vi "Read Speed Setting.vi"(8 "error in (no error)":errorcluster, 11 "Scientifica XYZ Gen1 in":refnum<class "Scientifica XYZ Gen1.lvclass">) -> (0 "error out":errorcluster, 1 "bytes read":u32, 2 "Speed Setting":string, 3 "Scientifica XYZ Gen1 out":refnum<class "Scientifica XYZ Gen1.lvclass">)   [LabVIEW 2020, in "TranslationStageClassStructure.lvlib" / "Scientifica XYZ Gen1.lvclass"]
uses:
  Scientifica XYZ Gen1.lvclass
  Scientifica XYZ Gen1.lvclass/Scientifica XYZ Gen1.ctl
  Serial Comms/Serial Comms/Serial Comms.lvclass
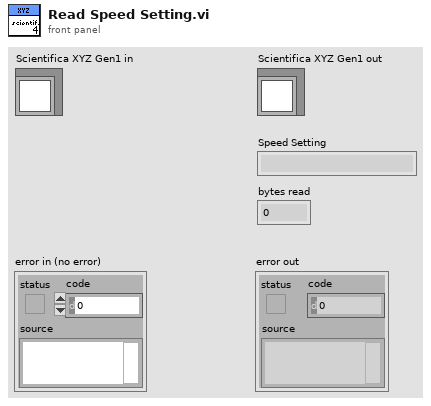
[diagram p1: front panel]
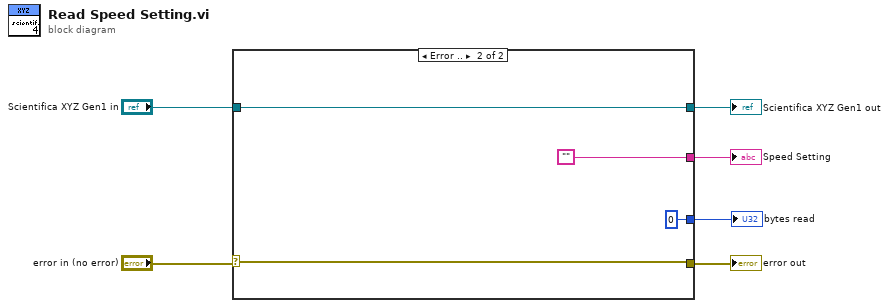
[diagram p0: block diagram]
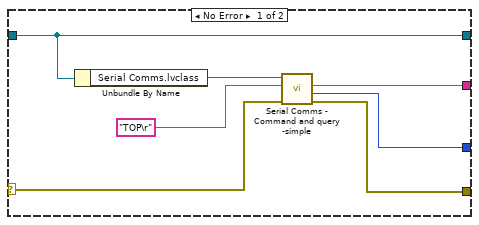
[diagram p2: hidden frame]
diagram:
  n1 = case shown="Error .." "error in (no error)" {
    selector: "error in (no error)" -> [w11 w16]
    tunnel: "Scientifica XYZ Gen1 in" -> [w13 w17]
    tunnel: [w13 w17] -> w4
    tunnel: [w10 w16] -> w3
    tunnel: [w8 ""] -> w2
    tunnel: [w7 u32 0 ("bytes read")] -> w1
    frame No Error {
      n2 = Unbundle By Name(w13) -> ("Serial Comms.lvclass"=w12:refnum<class "Serial Comms.lvclass">)
      n3 = call "Serial Comms - Command and query -simple.vi"("error in (no error)"=w11, "string to write"="TOP\r", "Serial Comms in"=w12) -> ("error out"=w10:errorcluster, "bytes read"=w7:u32, "read string"=w8:string)  [unwired: 4 in, 2 out]
    }
    frame Error {
    }
  }
  "error out" <- w3
  "Scientifica XYZ Gen1 out" <- w4
  "Speed Setting" <- w2
  "bytes read" <- w1
